vi "DT_Merge_Two Triangles.vi"(10 "Right Triangles":i32[][](array[numeric]), 11 "Left Triangles":i32[][](array[numeric])) -> (3 "Merged Triangles":i32[][](array[numeric]))   [LabVIEW 2020, in "NI_AAL_Geometry.lvlib"]
uses:
  <vilib>/Analysis/NI_AAL_Geometry.lvlib
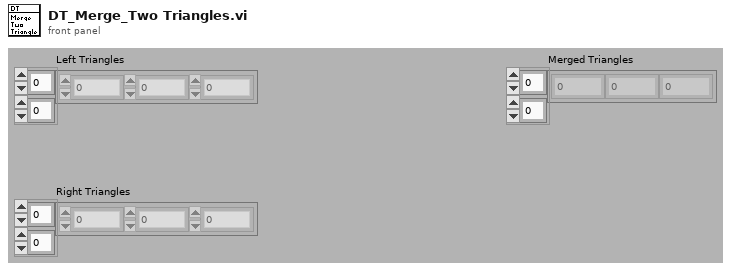
[diagram p1: front panel]
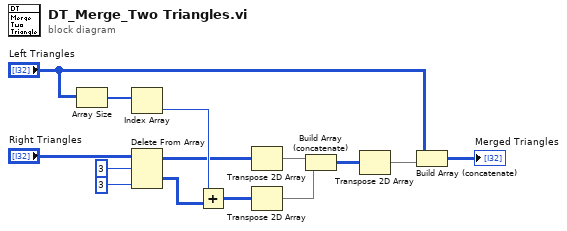
[diagram p0: block diagram]
diagram:
  n1 = Array Size(array="Left Triangles") -> (size(s)=w12:i32[])
  n2 = Index Array(array=w12) -> (element=w7:i32)  [unwired: 1 in]
  n3 = Delete From Array(array="Right Triangles", length=3, index (col)=3 ("disabled index (col)")) -> (deleted portion=w8:i32[][], array with subset deleted=w1:i32[][])  [unwired: 1 in]
  n4 = Add(x=w7, y=w8) -> (x+y=w6:i32[][])
  n5 = Transpose 2D Array(2D array=w1) -> (transposed array=w5:i32[][])
  n6 = Transpose 2D Array(2D array=w6) -> (transposed array=w4:i32[][])
  n7 = Build Array (concatenate)(w5, w4) -> (w3:i32[][])
  n8 = Transpose 2D Array(2D array=w3) -> (transposed array=w2:i32[][])
  n9 = Build Array (concatenate)("Left Triangles", w2) -> (→"Merged Triangles":i32[][])
